vi "Popup Template.vi"   [LabVIEW 2022 SP3, in "Audio Popup UI.lvlib"]
uses:
  Audio Popup UI.lvlib
panel:
  # "Use this as a starting point for popup dialogs"
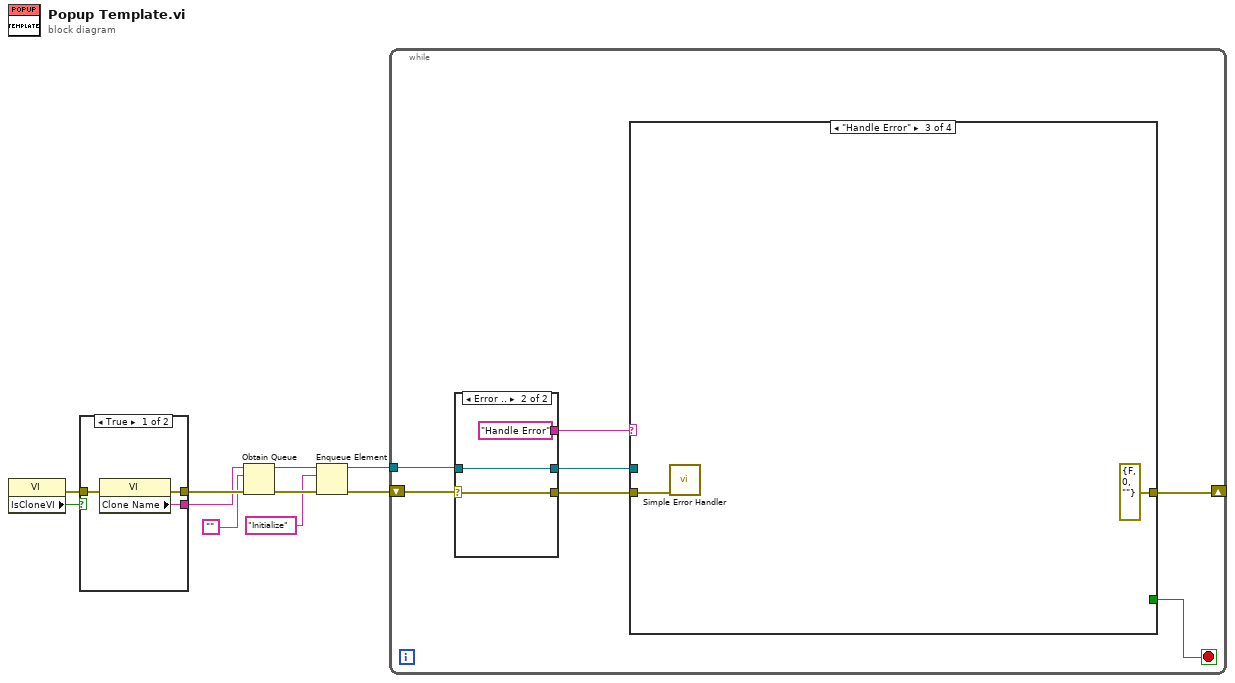
[diagram p0: block diagram]
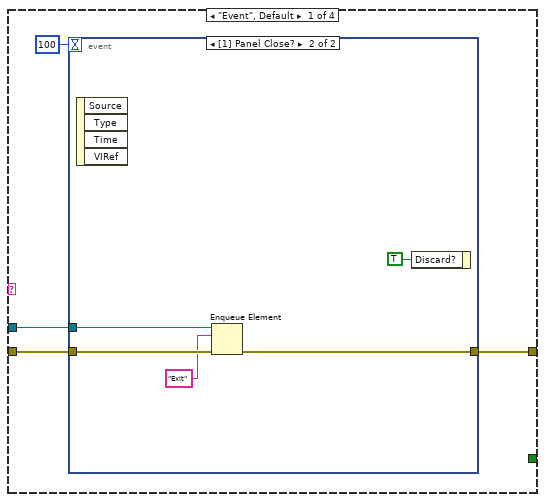
[diagram p2: hidden frame]
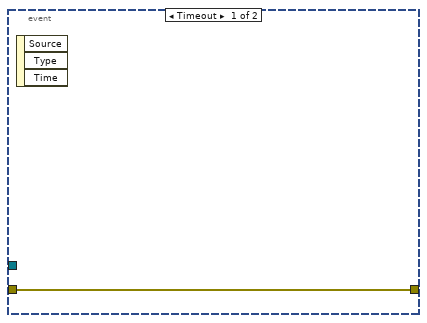
[diagram p3: hidden frame]
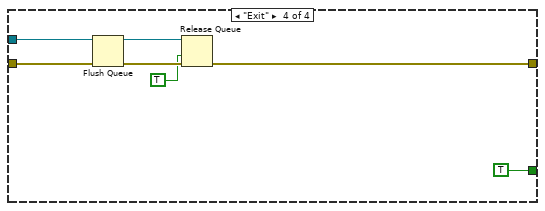
[diagram p5: hidden frame]
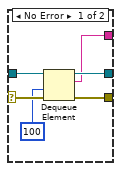
[diagram p6: hidden frame]
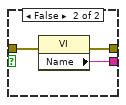
[diagram p7: hidden frame]
diagram:
  n1 = property class="VI"() -> (error out=w3:errorcluster, "IsCloneVI"=w4:bool)  [unwired: 2 in, 1 out]
  n2 = case shown="True" w4 {
    tunnel: [w13 w16] -> w10
    tunnel: [w12 w15] -> w9
    tunnel: w3 -> [w11 w14]
    frame True {
      n3 = property class="VI"(error in=w11) -> (error out=w13:errorcluster, "Clone Name"=w12:string)  [unwired: 1 in, 1 out]
    }
    frame False {
      n4 = property class="VI"(error in=w14) -> (error out=w16:errorcluster, "Name"=w15:string)  [unwired: 1 in, 1 out]
    }
  }
  n5 = Obtain Queue(name (unnamed)=w9, element data type="", error in (no error)=w10) -> (queue out=w7:refnum<queue>, error out=w8:errorcluster)  [unwired: 2 in, 1 out]
  n6 = Enqueue Element(queue=w7, element="Initialize", error in (no error)=w8) -> (queue out=w1:refnum<queue>, error out=w2:errorcluster)  [unwired: 1 in, 1 out]
  n7 = while {
    tunnel: w1 -> [w22]
    shift-right: [w18] -> _
    shift-left: w2 -> [w23]
    stop <- w17 stop-if-true
    n8 = case shown="Error .." w23 {
      selector: w23 -> [w49 w52]
      tunnel: [w48 w52] -> w19
      tunnel: w22 -> [w47 w51]
      tunnel: [w46 w51] -> w20
      tunnel: [w45 "Handle Error"] -> w21
      frame No Error {
        n9 = Dequeue Element(queue=w47, timeout in ms (-1)=100, error in (no error)=w49) -> (queue out=w46:refnum<queue>, element=w45:string, error out=w48:errorcluster)  [unwired: 1 out]
      }
      frame Error {
      }
    }
    n10 = case shown="\"Handle Error\"" w21 {
      tunnel: w20 -> [w25 _ _ w39]
      tunnel: w19 -> [w26 w34 w36 w40]
      tunnel: [w24 w34 errorcluster {"status"=FALSE, "code"=0, "source"=""} ("error out") w37] -> w18
      tunnel: [_ _ _ TRUE] -> w17
      frame "Event", Default {
        n11 = event shown="[1] Panel Close?" {
          selector: _ -> [_ _]
          dyn-events: _ -> [_ _]
          timeout: 100 -> [_ _]
          tunnel: w26 -> [w28 w32]
          tunnel: w25 -> [_ w31]
          tunnel: [w28 w29] -> w24
          event Timeout {
            n12 = event-data() -> ()  [unwired: 1 in, 3 out]
          }
          event Panel Close? {
            n13 = event-data() -> ()  [unwired: 1 in, 4 out]
            n14 = Enqueue Element(queue=w31, element="Exit", error in (no error)=w32) -> (error out=w29:errorcluster)  [unwired: 1 in, 2 out]
            n15 = event-data("Discard?"=TRUE) -> ()  [unwired: 1 in, 1 out]
          }
        }
      }
      frame "Initialize" {
      }
      frame "Handle Error" {
        n16 = call <vilib>:"Simple Error Handler.vi"("error in (no error)"=w36) -> ()  [unwired: 4 in, 5 out]
      }
      frame "Exit" {
        n17 = Flush Queue(queue=w39, error in (no error)=w40) -> (queue out=w43:refnum<queue>, error out=w42:errorcluster)  [unwired: 1 out]
        n18 = Release Queue(queue=w43, force destroy? (F)=TRUE, error in (no error)=w42) -> (error out=w37:errorcluster)  [unwired: 2 out]
      }
    }
  }
